vi "CAN Global.vi"(0 "Controller Type:":T2, 2 "Write (F)":bool, 5 "CAN Cmd":dbl, 7 "Power Relay":T1, 9 "Ignition Relay":T1) -> (4 "Controller Type OUT":T2, 6 "CAN Cmd OUT":dbl, 8 "Power Relay OUT":T1, 10 "Ignition Relay OUT":T1)   [LabVIEW 2019]
uses:
  Type Defs/Controller Names.ctl
panel:
  out "CAN CMD":dbl
  in  "Controller Type:":T2
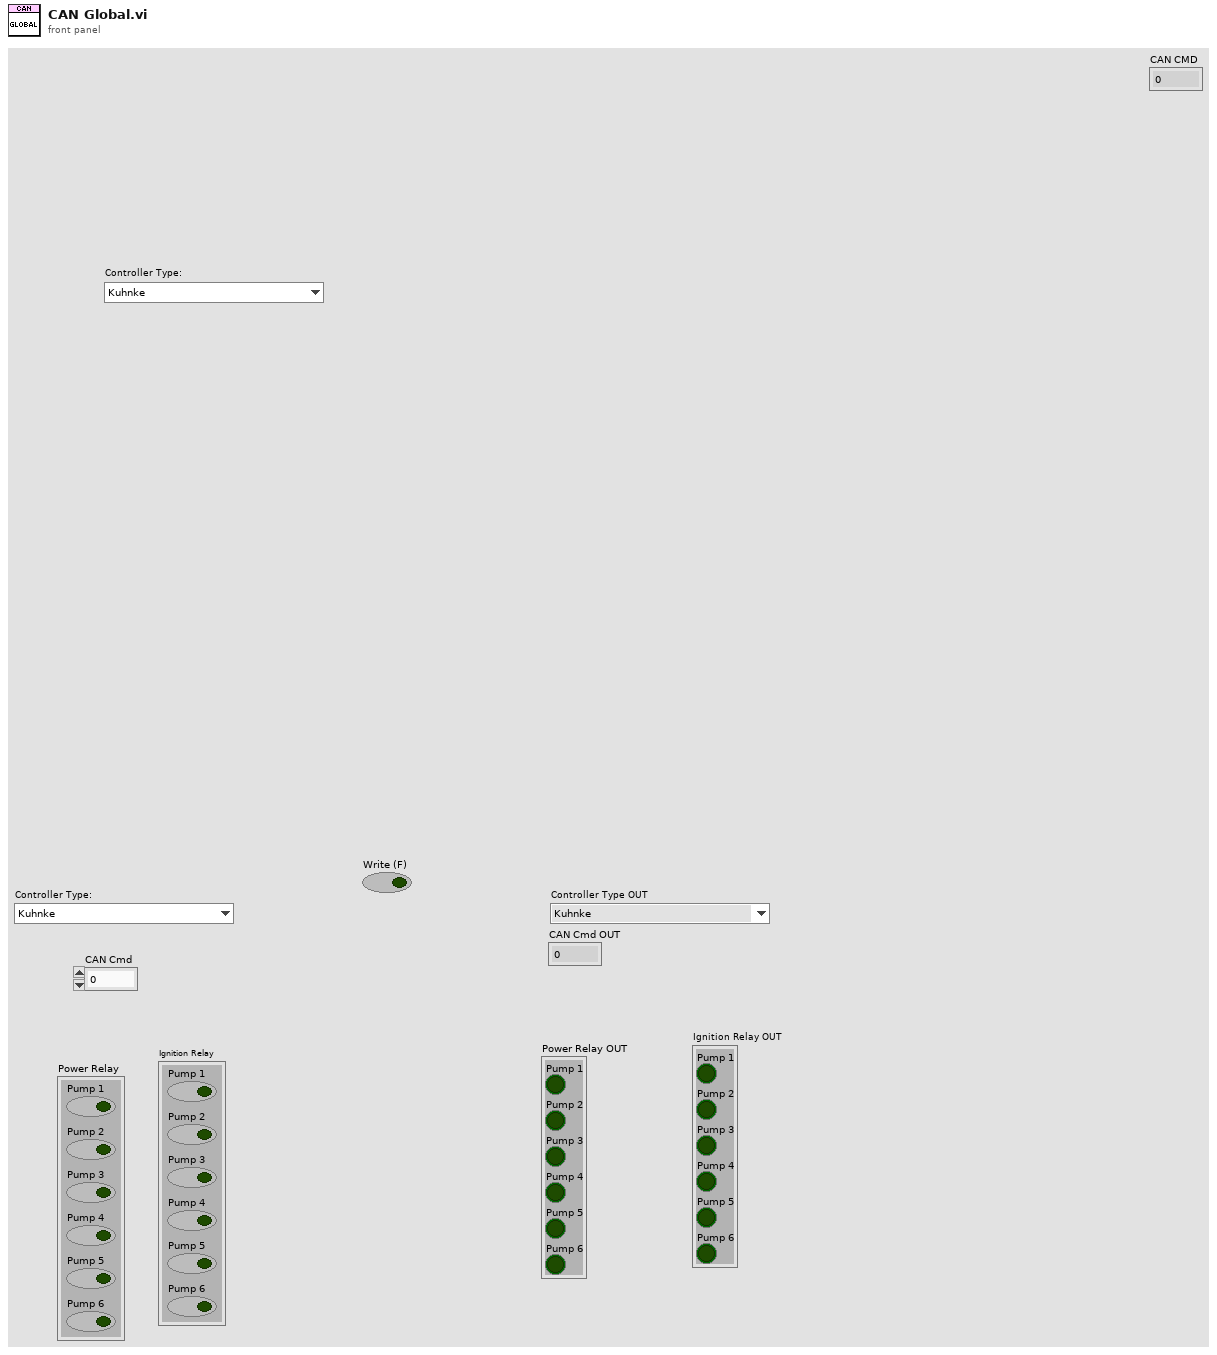
[diagram p1: front panel]
types:
  T1 = cluster{"Pump 1":bool, "Pump 2":bool, "Pump 3":bool, "Pump 4":bool, "Pump 5":bool, "Pump 6":bool}
  T2 = typedef "Controller Names.ctl" = enum16{"Kuhnke", "Helbako BLDC", "Conti", "Hella BLDC OL PWM", "Hella BLDC Turbine OL PWM", "Hella BLDC Pressure", "Helbako (old)", "TI PWM", "PSA", "Hella Gas", "Hella Diesel", "8 Comm", "10 Comm", "8 Comm Hella", "10 Comm Hella", "8 Comm Omron", "10 Comm Omron", "8 Comm Nissan", "10 Comm Nissan", "8 Comm Hella (for FCA)", "Mazda BLDC"}
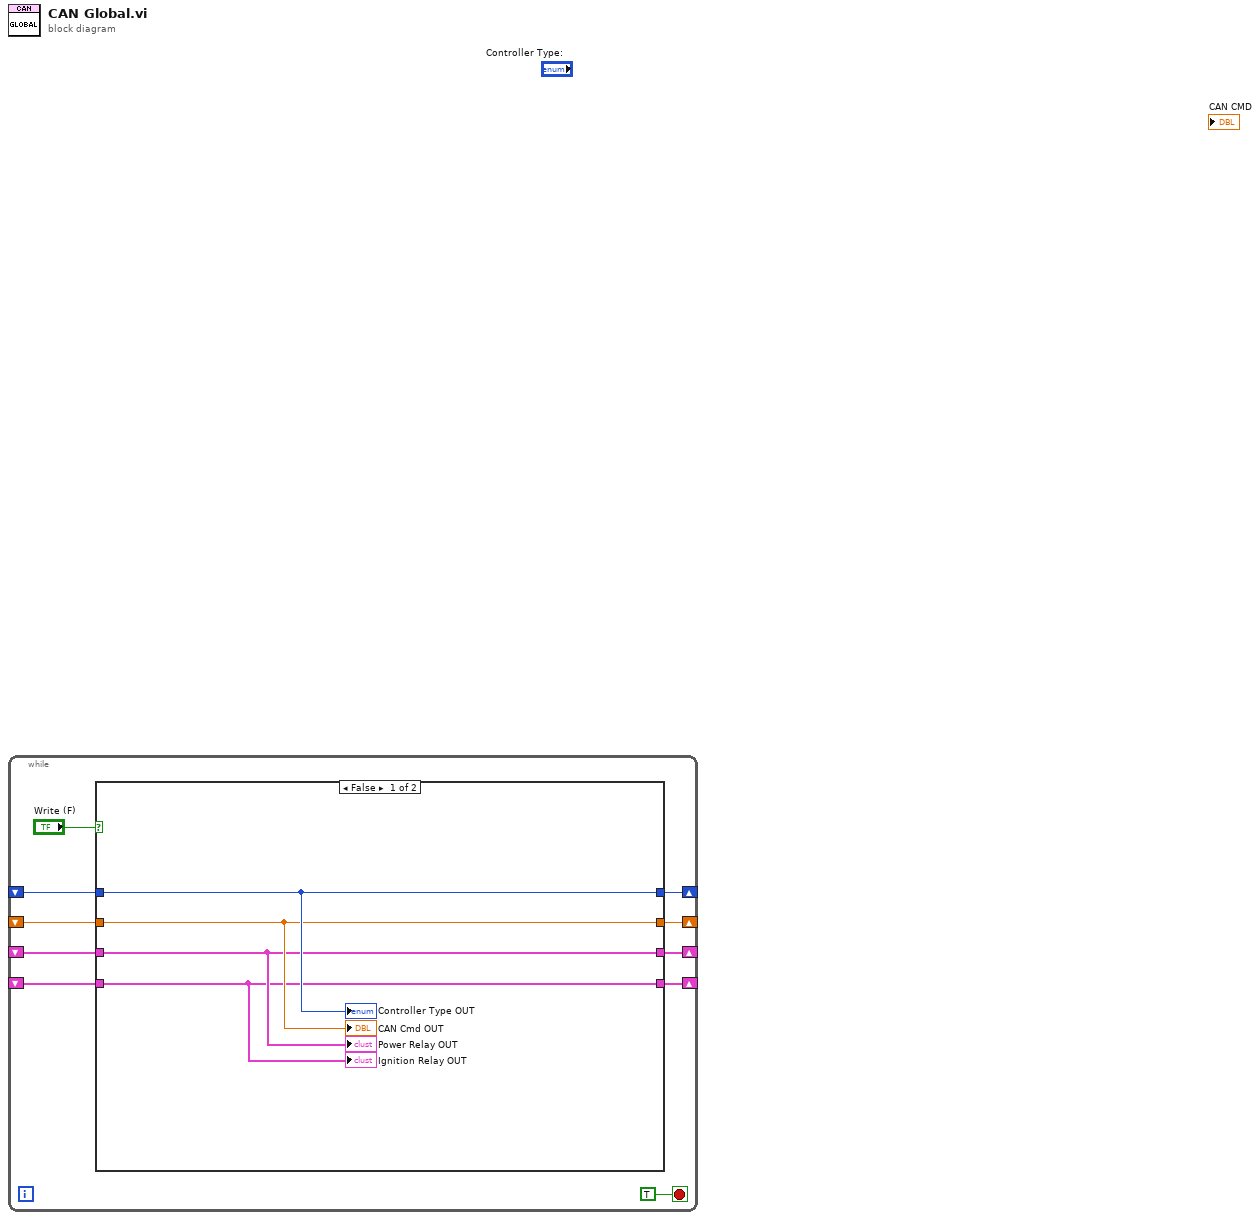
[diagram p0: block diagram]
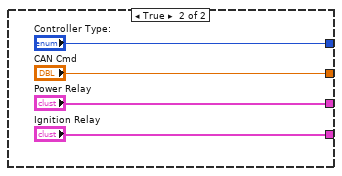
[diagram p2: hidden frame]
diagram:
  n1 = while {
    shift-right: [w8] -> _
    shift-left: _ -> [w5]
    shift-right: [w7] -> _
    shift-left: _ -> [w4]
    shift-right: [w6] -> _
    shift-left: _ -> [w3]
    shift-right: [w2] -> _
    shift-left: _ -> [w1]
    stop <- TRUE stop-if-true
    n2 = case shown="False" "Write (F)" {
      tunnel: [w14 "Controller Type:"] -> w8
      tunnel: [w13 "CAN Cmd"] -> w7
      tunnel: [w12 "Power Relay"] -> w6
      tunnel: w5 -> [w14 _]
      tunnel: w4 -> [w13 _]
      tunnel: w3 -> [w12 _]
      tunnel: [w11 "Ignition Relay"] -> w2
      tunnel: w1 -> [w11 _]
      frame False {
        "Controller Type OUT" <- w14
        "CAN Cmd OUT" <- w13
        "Power Relay OUT" <- w12
        "Ignition Relay OUT" <- w11
      }
      frame True {
      }
    }
  }
